vi "FF_StaightLinePath.vi"(8 "error in (no error)":errorcluster, 9 "WristVelocity":dbl[](array[numeric]), 10 "WristPosition":dbl[](array[numeric]), 11 "Force Field Controller in":refnum<class "ForceField.lvclass">) -> (0 "error out":errorcluster, 1 "ClosestPt":dbl[](array[numeric]), 2 "Force":dbl[](array[numeric]), 3 "Force Field Controller out":refnum<class "ForceField.lvclass">, 4 "ForceComp":dbl[](array[numeric]))   [LabVIEW 2016, in "ForceField.lvclass"]
uses:
  ForceField.lvclass
  ForceField.lvclass/ForceField.ctl
  TypeDef/TND.ctl
  <vilib>/Analysis/BLAS.llb/dnrm2 - Vector 2-Norm (DBL).vi
  <vilib>/ptbypt/NI_PtbyPt.lvlib
  <vilib>/Analysis/NI_AALBLAS.lvlib
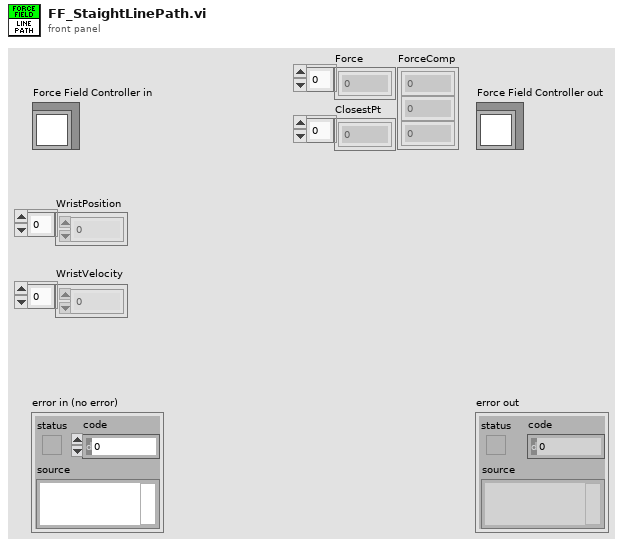
[diagram p1: front panel]
types:
  T1 = typedef "ForceField.lvclass/TND.ctl" = cluster{"Vt":dbl[], "Vn":dbl[], "Dmin":dbl}
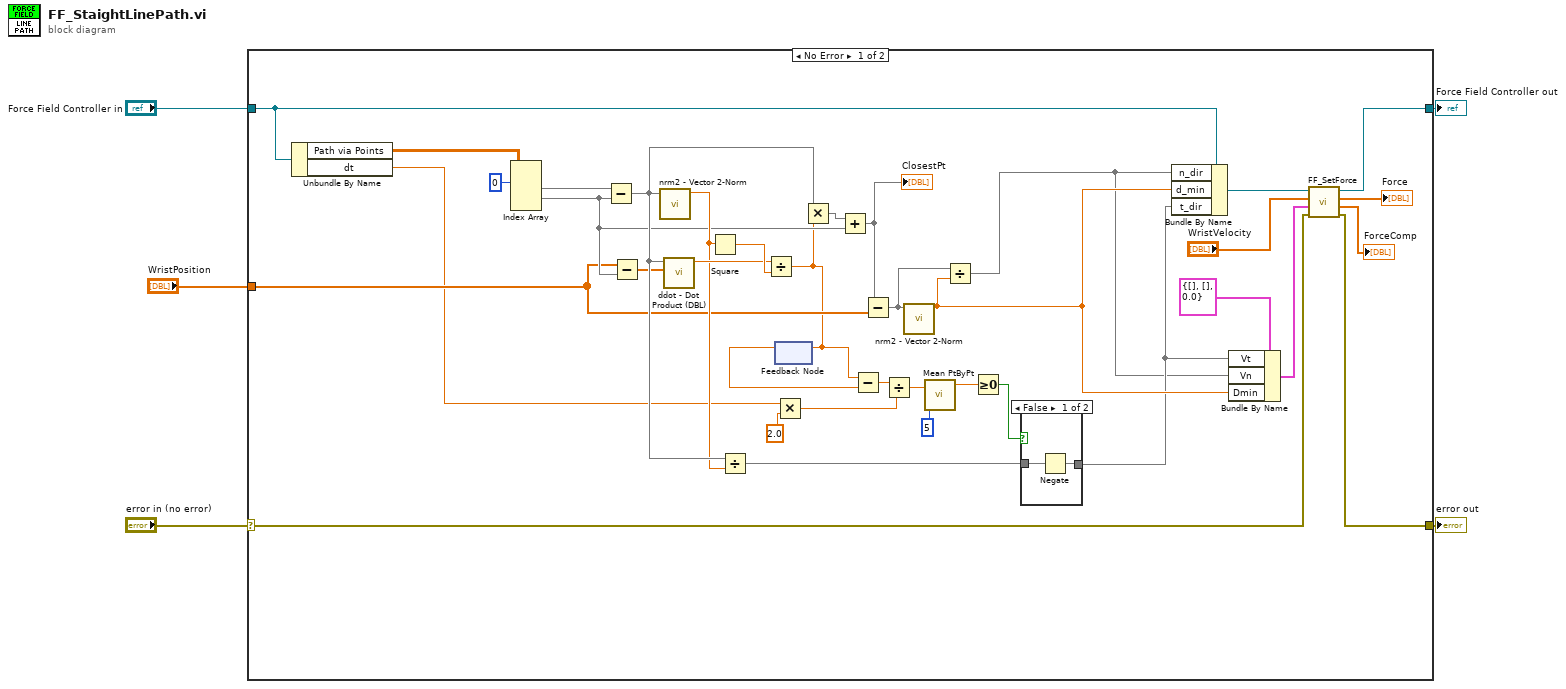
[diagram p0: block diagram]
diagram:
  n1 = case shown="No Error" "error in (no error)" {
    selector: "error in (no error)" -> [w15 w47]
    tunnel: [w14 w47] -> w4
    tunnel: [w17 w46] -> w2
    tunnel: "Force Field Controller in" -> [w20 w46]
    tunnel: "WristPosition" -> [w30 _]
    frame No Error {
      n2 = Unbundle By Name(w20) -> ("Path via Points"=w34:dbl[][], "dt"=w25:dbl)
      n3 = Index Array(array=w34, index (row) #1=0 ("index (row)")) -> (element #1=w32:dbl[], element #2=w31:dbl[])  [unwired: 3 in]
      n4 = Subtract(x=w32, y=w31) -> (x-y=w42:dbl[])
      n5 = Subtract(x=w30, y=w31) -> (x-y=w41:dbl[])
      n6 = call-poly <vilib>:"nrm2 - Vector 2-Norm.vi"("x"=w42) -> ("dnrm2"=w36:dbl)  [unwired: 9 in, 1 out]
      n7 = call <vilib>:"ddot - Dot Product (DBL).vi"("y"=w41, "x"=w42) -> ("ddot"=w39:dbl)  [unwired: 8 in, 1 out]
      n8 = Square(x=w36) -> (x^2=w40:dbl)
      n9 = Divide(x=w42, y=w36) -> (x/y=w23:dbl[])
      n10 = Divide(x=w39, y=w40) -> (x/y=w19:dbl)
      n11 = feedback-in #1(w19) -> ()
      n12 = feedback #1() -> (w12:dbl)  [unwired: 1 in]
      n13 = Multiply(x=w25, y=2.0) -> (x*y=w24:dbl)
      n14 = Multiply(x=w42, y=w19) -> (x*y=w38:dbl[])
      n15 = Add(x=w38, y=w31) -> (x+y=w37:dbl[])
      "ClosestPt" <- w37
      n16 = Subtract(x=w19, y=w12) -> (x-y=w29:dbl)
      n17 = Subtract(x=w37, y=w30) -> (x-y=w35:dbl[])
      n18 = Divide(x=w29, y=w24) -> (x/y=w28:dbl)
      n19 = call-poly <vilib>:"nrm2 - Vector 2-Norm.vi"("x"=w35) -> ("dnrm2"=w8:dbl)  [unwired: 9 in, 1 out]
      n20 = call <vilib>:"Mean PtByPt.vi"("x"=w28, "sample length"=5) -> ("mean"=w22:dbl)  [unwired: 2 in, 1 out]
      n21 = Divide(x=w35, y=w8) -> (x/y=w6:dbl[])
      n22 = Greater Or Equal To 0?(x=w22) -> (x >= 0?=w21:bool)
      n23 = case shown="False" w21 {
        tunnel: w23 -> [w44 w45]
        tunnel: [w43 w45] -> w7
        frame False {
          n24 = Negate(x=w44) -> (-x=w43:dbl[])
        }
        frame True {
        }
      }
      n25 = Bundle By Name(cluster=w20, "n_dir"=w6, "d_min"=w8, "t_dir"=w7) -> (w18:refnum<class "ForceField.lvclass">)
      n26 = Bundle By Name(cluster=T1 {"Vt"=[], "Vn"=[], "Dmin"=0.0} ("TND"), "Vt"=w7, "Vn"=w6, "Dmin"=w8) -> (w9:T1)
      n27 = call "FF_SetForce.vi"("error in (no error)"=w15, "TND"=w9, "AnkleVelocity"="WristVelocity", "Force Field Controller in"=w18) -> ("error out"=w14:errorcluster, "ForceNTD"=→"ForceComp":dbl[], "ForceXYZ"=→"Force":dbl[], "Force Field Controller out"=w17:refnum<class "ForceField.lvclass">)  [unwired: 4 in]
    }
    frame Error {
    }
  }
  "error out" <- w4
  "Force Field Controller out" <- w2
